vi "Leaderboard export March.vi"(9 "Time Stamp":timestamp, 11 "path to PNG file":path) -> (0 "error out":errorcluster, 3 "path":path)   [LabVIEW 2020, in "Visualisation.lvclass"]
uses:
  Visualisation.lvclass
  Application/Globals.vi
  Data Manager/Data Manager.lvclass
  Application/Application.lvlib
panel:
  in  "Export":enum32{"Page 1", "Page 2"}(tab)
  out "Run":T1(array[cluster]) {"Distance 2" scale=0.0..32.7792}
  out "Walk":T1(array[cluster]) {"Distance 2" scale=0.0..14.5509}
  out "Table Control":string[][](table)
  out "Total Travelled":dbl format="%0.1f km"
  out "Days":dbl format="Day: %d"
  out "Leaderboard":T2(array[cluster]) {"Distance" scale=0.0..40.06335}
  # "Longest Single Activity"
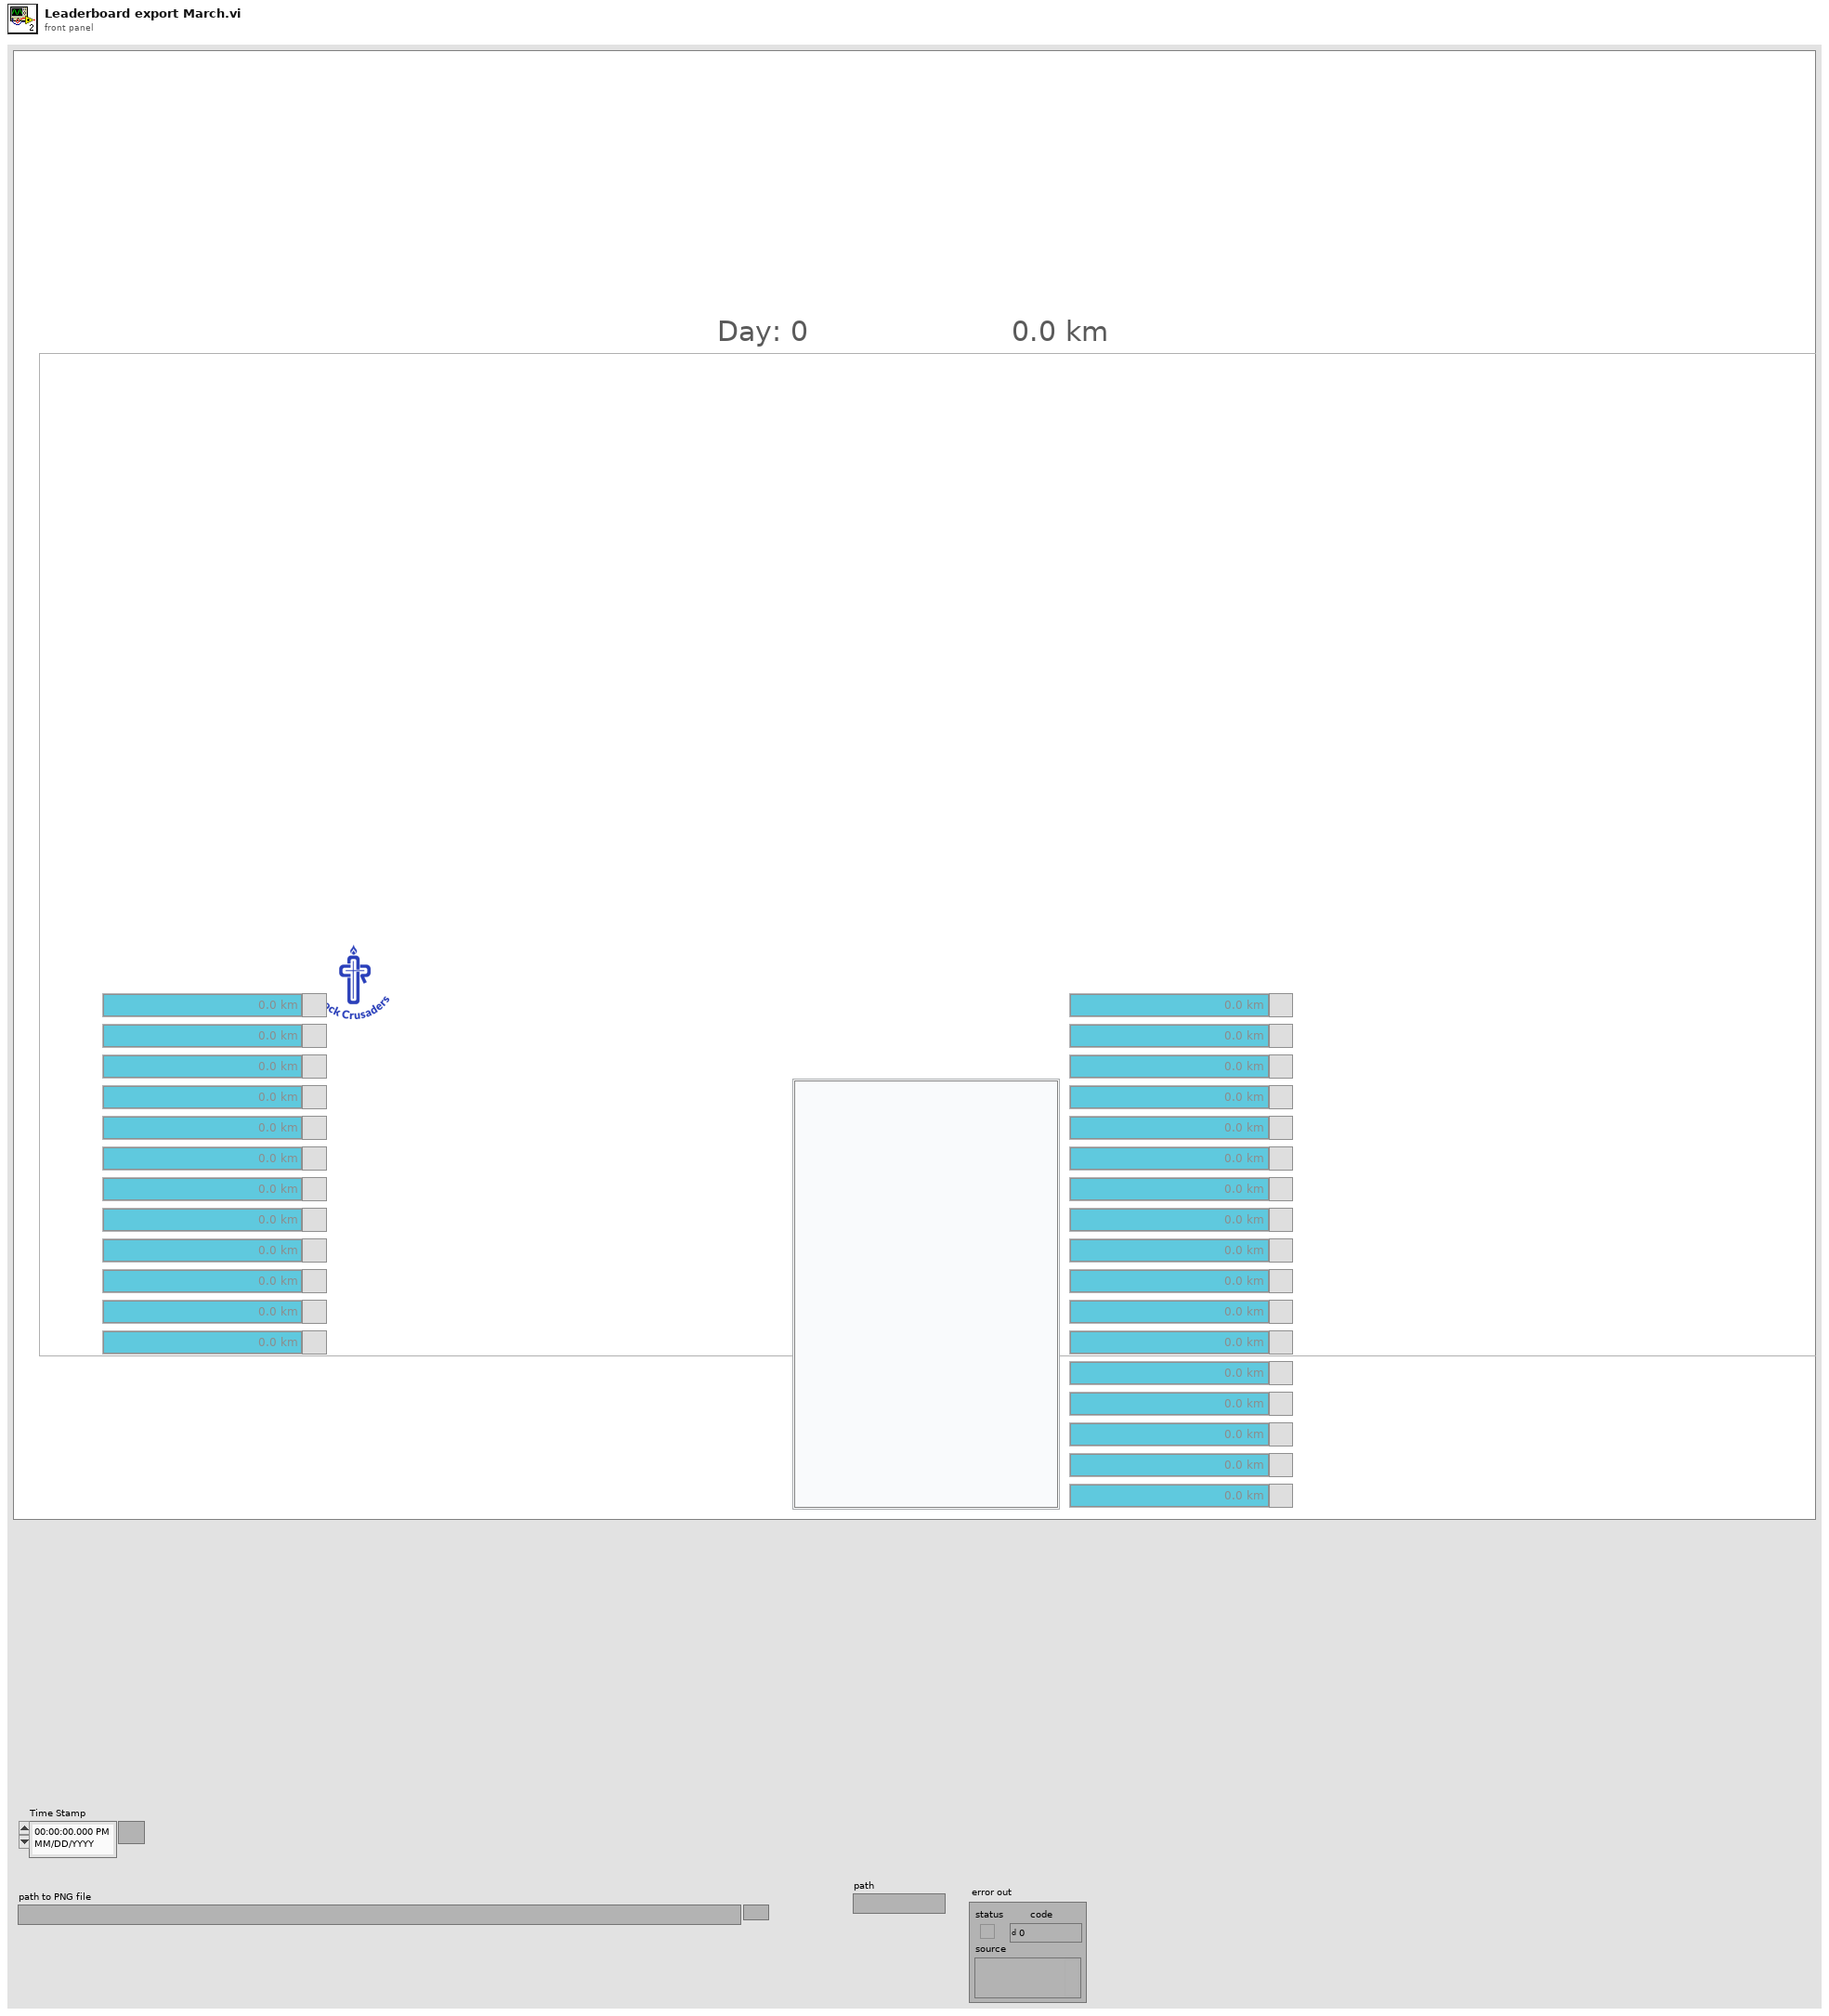
[diagram p1: front panel]
types:
  T1 = cluster{"Athlete":string, "Team":u32, "Distance 2":dbl}[]
  T2 = cluster{"Athlete":string, "Distance":dbl, "Team":u32}[]
  T3 = cluster{"Athlete":string, "Distance":dbl, "Team":u32}
  T4 = cluster{"Athlete":string, "Team":u32, "Distance 2":dbl}
  T5 = typedef "LVDateTimeRec.ctl" = cluster{"fractional second":dbl, "second":i32, "minute":i32, "hour":i32, "day of month":i32, "month":i32, "year":i32, "day of week":i32, "day of year":i32, "DST":i32}
  T6 = cluster{"Athlete":string, "Distance":dbl, "Team":u32, "Distance 2":cluster{"Numeric":dbl, "Numeric":dbl, "Numeric":dbl}}
  T7 = typedef "imagedata.ctl" = cluster{"image type":i32, "image depth":i32, "image":u8[], "mask":u8[], "colors":u32[], "Rectangle":cluster{"left":i16, "top":i16, "right":i16, "bottom":i16}}
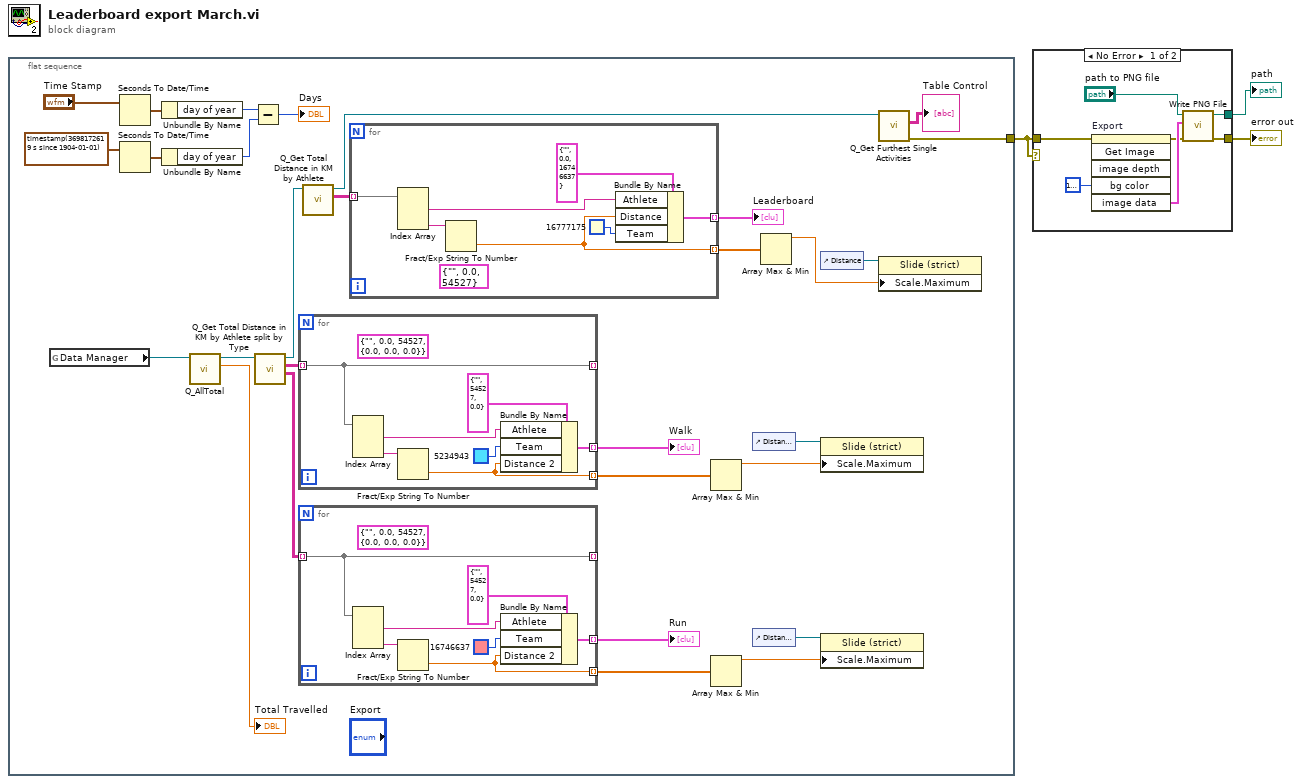
[diagram p0: block diagram]
diagram:
  n1 = flat-sequence {
    tunnel: [w14] -> w1
    frame #0 {
      n2 = global read "Globals.vi" "Data Manager"() -> (w6:refnum<class "Data Manager.lvclass">)
      n3 = Seconds To Date/Time(time stamp (now)="Time Stamp") -> (date time rec=w11:T5)  [unwired: 1 in]
      n4 = Seconds To Date/Time(time stamp (now)=timestamp(3698172619.613 s since 1904-01-01) ("Time Stamp")) -> (date time rec=w12:T5)  [unwired: 1 in]
      n5 = Unbundle By Name(w11) -> ("day of year"=w9:i32)
      n6 = Unbundle By Name(w12) -> ("day of year"=w8:i32)
      n7 = call-dynamic "Q_AllTotal.vi"("Data Manager in"=w6) -> ("Total Travelled"=→"Total Travelled":dbl, "Data Manager out"=w5:refnum<class "Data Manager.lvclass">)  [unwired: 7 in, 2 out]
      n8 = Subtract(x=w9, y=w8) -> (x-y=→"Days":i32)
      n9 = call-dynamic "Q_Get Total Distance in KM by Athlete split by Type.vi"("Data Manager in"=w5) -> ("Run"=w27:string[][], "Walk"=w31:string[][], "Data Manager out"=w24:refnum<class "Data Manager.lvclass">)  [unwired: 6 in, 2 out]
      n10 = for {
        tunnel: [w50] -> _ mode=indexing
        tunnel: [w53] -> w18 mode=indexing
        tunnel: w31 -> [w50] mode=indexing
        tunnel: [w49] -> w28 mode=indexing
        (unwired) T6 {"Athlete"="", "Distance"=0.0, "Team"=54527, "Distance 2"={"Numeric"=0.0, "Numeric"=0.0, "Numeric"=0.0}} ("Leaderboard")
        n11 = Index Array(array=w50) -> (element #1=w51:string, element #3=w52:string)  [unwired: 3 in, 1 out]
        n12 = Fract/Exp String To Number(string=w52) -> (number=w49:dbl)  [unwired: 3 in, 1 out]
        n13 = Bundle By Name(cluster=T4 {"Athlete"="", "Team"=54527, "Distance 2"=0.0} ("Leaderboard"), "Athlete"=w51, "Team"=u32 5234943 ("Color Box"), "Distance 2"=w49) -> (w53:T4)
      }
      "Walk" <- w18
      n14 = for {
        tunnel: w27 -> [w43] mode=indexing
        tunnel: [w46] -> w25 mode=indexing
        tunnel: [w43] -> _ mode=indexing
        tunnel: [w42] -> w26 mode=indexing
        (unwired) T6 {"Athlete"="", "Distance"=0.0, "Team"=54527, "Distance 2"={"Numeric"=0.0, "Numeric"=0.0, "Numeric"=0.0}} ("Leaderboard")
        n15 = Index Array(array=w43) -> (element #1=w44:string, element #3=w45:string)  [unwired: 3 in, 1 out]
        n16 = Fract/Exp String To Number(string=w45) -> (number=w42:dbl)  [unwired: 3 in, 1 out]
        n17 = Bundle By Name(cluster=T4 {"Athlete"="", "Team"=54527, "Distance 2"=0.0} ("Leaderboard"), "Athlete"=w44, "Team"=u32 16746637 ("Color Box"), "Distance 2"=w42) -> (w46:T4)
      }
      "Run" <- w25
      n18 = call-dynamic "Q_Get Total Distance in KM by Athlete.vi"("Data Manager in"=w24) -> ("Result Set"=w23:string[][], "Data Manager out"=w15:refnum<class "Data Manager.lvclass">)  [unwired: 8 in, 1 out]
      n19 = for {
        tunnel: w23 -> [w38] mode=indexing
        tunnel: [w39] -> w22 mode=indexing
        tunnel: [w34] -> w20 mode=indexing
        (unwired) T3 {"Athlete"="", "Distance"=0.0, "Team"=54527} ("Leaderboard")
        n20 = Index Array(array=w38) -> (element #1=w36:string, element #3=w37:string)  [unwired: 3 in, 1 out]
        n21 = Fract/Exp String To Number(string=w37) -> (number=w34:dbl)  [unwired: 3 in, 1 out]
        n22 = Bundle By Name(cluster=T3 {"Athlete"="", "Distance"=0.0, "Team"=16746637} ("Leaderboard"), "Athlete"=w36, "Distance"=w34, "Team"=u32 16777175 ("Color Box")) -> (w39:T3)
      }
      "Leaderboard" <- w22
      n23 = Array Max & Min(array=w28) -> (max value=w29:dbl)  [unwired: 3 out]
      n24 = Array Max & Min(array=w26) -> (max value=w32:dbl)  [unwired: 3 out]
      n25 = control-ref of="Distance 2"() -> (w30:refnum<vi>)
      n26 = control-ref of="Distance 2"() -> (w17:refnum<vi>)
      n27 = Array Max & Min(array=w20) -> (max value=w21:dbl)  [unwired: 3 out]
      n28 = control-ref of="Distance"() -> (w19:refnum<vi>)
      n29 = property on="Property Node" class="Slide (strict)"(reference=w30, "Scale.Maximum"=w29) -> ()  [unwired: 1 in, 2 out]
      n30 = property on="Property Node" class="Slide (strict)"(reference=w17, "Scale.Maximum"=w32) -> ()  [unwired: 1 in, 2 out]
      n31 = call-dynamic "Q_Get Furthest Single Activities.vi"("Data Manager in"=w15) -> ("error out"=w14:errorcluster, "Result Set"=→"Table Control":string[][])  [unwired: 8 in, 1 out]
      n32 = property on="Property Node" class="Slide (strict)"(reference=w19, "Scale.Maximum"=w21) -> ()  [unwired: 1 in, 2 out]
    }
  }
  n33 = case shown="No Error" w1 {
    tunnel: w1 -> [w58 _]
    tunnel: [w56 _] -> w3
    tunnel: [w55 _] -> w2
    frame No Error {
      n34 = invoke on="Export" class="TabCtl (strict)" method="Get Image"(error in=w58, "bg color"=u32 16777216 ("Background Color")) -> (error out=w54:errorcluster, "image data"=w59:T7)  [unwired: 4 in, 4 out]
      n35 = call <vilib>:"Write PNG File.vi"("error in (no error)"=w54, "image data"=w59, "path to PNG file"="path to PNG file") -> ("error out"=w55:errorcluster, "path"=w56:path)  [unwired: 7 in]
    }
    frame Error {
    }
  }
  "path" <- w3
  "error out" <- w2
